vi "Set Timeout.vi"(8 "Error In":errorcluster, 10 "Timeout (s)":i32=10000, 11 "OPI Ref":refnum<data-value>) -> (0 "Error Out":errorcluster, 3 "OPI Ref":refnum<data-value>)   [LabVIEW 2016, in "OPI.lvclass"]
doc: "Set the timeout for localhost communication with Python Execution Server. Default timeout is 10s. In some cases this might be to little for functions that take longer to execute. In such case using this method can resolve the problem of waiting longer."
uses:
  OPI.lvclass
  OPI.lvclass/OPI.ctl
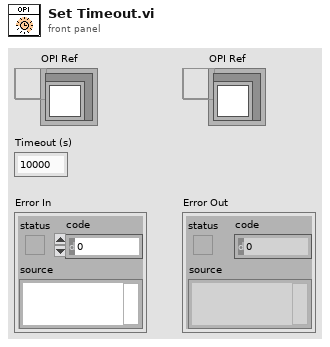
[diagram p1: front panel]
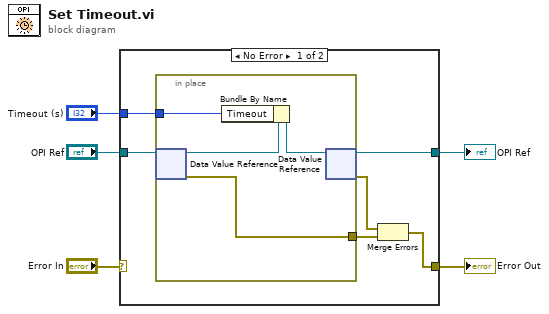
[diagram p0: block diagram]
diagram:
  n1 = case shown="No Error" "Error In" {
    selector: "Error In" -> [_ w16]
    tunnel: "OPI Ref" -> [w11 w17]
    tunnel: [w10 w17] -> w4
    tunnel: [w7 w16] -> w2
    tunnel: "Timeout (s)" -> [w6 _]
    frame No Error {
      n2 = in-place {
        in-place-border: [w13] -> w8
        in-place-border: w6 -> [w12]
        n3 = in-place-dvr #1(w11) -> (w14:refnum<class "OPI.lvclass">, w13:errorcluster)
        n4 = Bundle By Name(cluster=w14, "Timeout"=w12) -> (w15:refnum<class "OPI.lvclass">)
        n5 = in-place-dvr #1(w15) -> (w10:refnum<data-value>, w9:errorcluster)
      }
      n6 = Merge Errors(w9, w8) -> (w7:errorcluster)
    }
    frame Error {
    }
  }
  "Error Out" <- w2
  "OPI Ref" <- w4
